vi "GenerateLab.vi"(8 "ROI":T1, 9 "Lighting":u16(ring)=5 items=["Incandescent/tungsten", "Old direct sunlight at noon", "Old daylight", "ICC profile PCS", "Mid-morning daylight", "Daylight, sRGB, Adobe-RGB", "North sky daylight", "Equal energy", "Daylight Fluorescent", "Cool fluorescent", "White Fluorescent", "Warm White Fluorescent", "Daylight Fluorescent", "Lite White Fluorescent", "Daylight fluorescent, D65 simulator", "Sylvania F40, D50 simulator", "Cool White Fluorescent", "Ultralume 50, Philips TL85", "Ultralume 40, Philips TL84", "Ultralume 30, Philips TL83"], 11 "image data":T2) -> (1 "Dimensions":string, 3 "Plots":T3)   [LabVIEW 2020]
uses:
  <vilib>/picture/picture.llb/imagedata.ctl
panel:
  out "b":dbl[](graph)
  out "a":dbl[](graph)
  out "L":dbl[](graph)
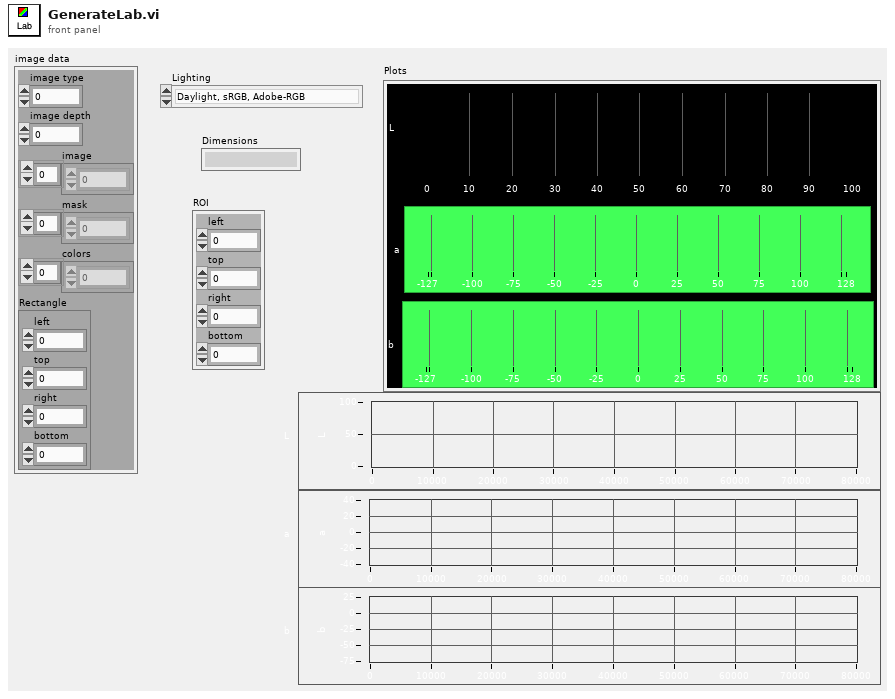
[diagram p1: front panel]
types:
  T1 = cluster{"left":i32, "top":i32, "right":i32, "bottom":i32}
  T2 = typedef "imagedata.ctl" = cluster{"image type":i32, "image depth":i32, "image":u8[], "mask":u8[], "colors":u32[], "Rectangle":cluster{"left":i16, "top":i16, "right":i16, "bottom":i16}}
  T3 = cluster{"L":dbl[], "a":cluster{i32, i32, dbl[]}, "b":cluster{i32, i32, dbl[]}}
  T4 = cluster{dbl[], cluster{i32, i32, dbl[]}, cluster{i32, i32, dbl[]}}
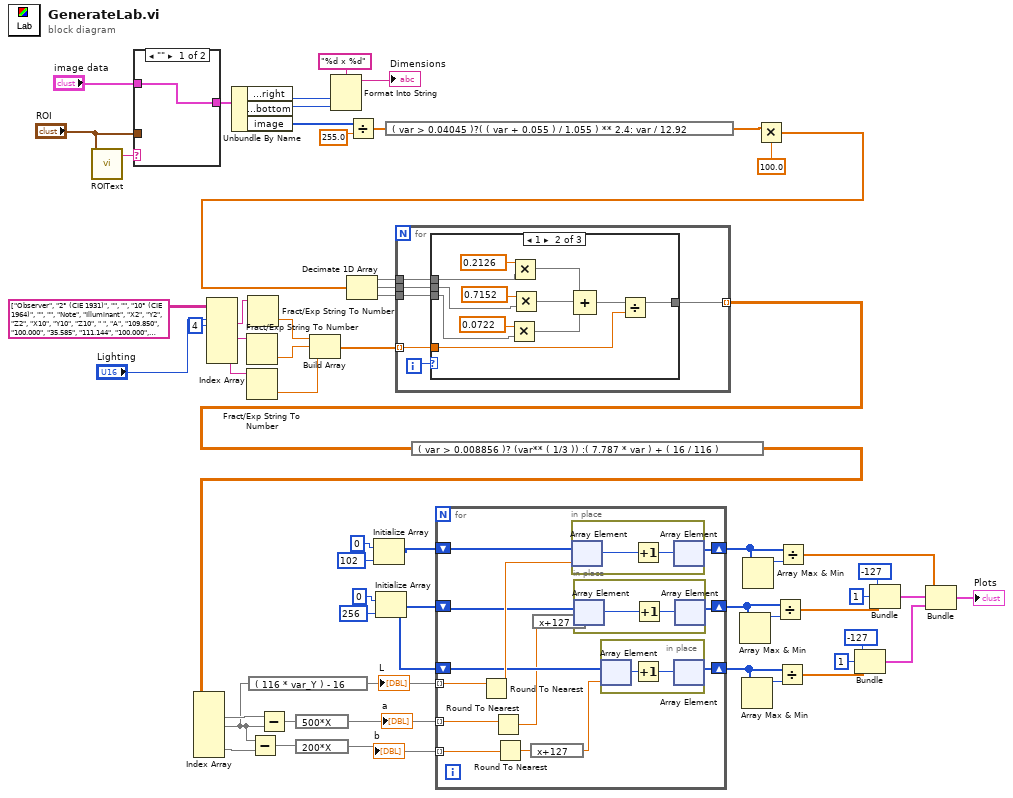
[diagram p0: block diagram]
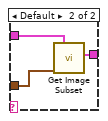
[diagram p2: hidden frame]
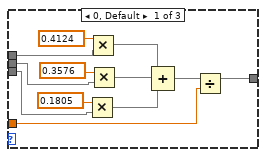
[diagram p3: hidden frame]
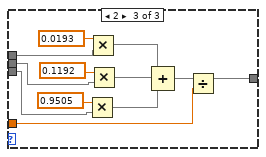
[diagram p4: hidden frame]
diagram:
  n1 = call "ROIText.vi"("ROI"="ROI") -> ("r"=w1:string)  [unwired: 7 in, 3 out]
  n2 = case shown="\"\"" w1 {
    tunnel: "image data" -> [w60 w63]
    tunnel: [w60 w62] -> w3
    tunnel: "ROI" -> [_ w61]
    frame "" {
    }
    frame Default {
      n3 = call <vilib>:"Get Image Subset.vi"("subset rect"=w61, "image data"=w63) -> ("image subset"=w62:T2)  [unwired: 4 in, 1 out]
    }
  }
  n4 = Index Array(array=string[][] [["Observer", "2° (CIE 1931)", "", "", "10° (CIE 1964)", "", "", "Note"], ["Illuminant", "X2", "Y2", "Z2", "X10", "Y10", "Z10", " "], ["A", "109.850", "100.000", "35.585", "111.144", "100.000", "35.200", "Incandescent/tungsten"], ["B", "99.0927", "100.000", "85.313", "99.178;", "100.000", "84.3493", "Old direct sunlight at noon"], ["C", "98.074", "100.000", "118.232", "97.285", "100.000", "116.145", "Old daylight"], ["D50", "96.422", "100.000", "82.521", "96.720", "100.000", "81.427", "ICC profile PCS"], ["D55", "95.682", "100.000", "92.149", "95.799", "100.000", "90.926", "Mid-morning daylight"], ["D65", "95.047", "100.000", "108.883", "94.811", "100.000", "107.304", "Daylight, sRGB, Adobe-RGB"], ["D75", "94.972", "100.000", "122.638", "94.416", "100.000", "120.641", "North sky daylight"], ["E", "100.000", "100.000", "100.000", "100.000", "100.000", "100.000", "Equal energy"], ["F1", "92.834", "100.000", "103.665", "94.791", "100.000", "103.191", "Daylight Fluorescent"], ["F2", "99.187", "100.000", "67.395", "103.280", "100.000", "69.026", "Cool fluorescent"], ["F3", "103.754", "100.000", "49.861", "108.968", "100.000", "51.965", "White Fluorescent"], ["F4", "109.147", "100.000", "38.813", "114.961", "100.000", "40.963", "Warm White Fluorescent"], ["F5", "90.872", "100.000", "98.723", "93.369", "100.000", "98.636", "Daylight Fluorescent"], ["F6", "97.309", "100.000", "60.191", "102.148", "100.000", "62.074", "Lite White Fluorescent"], ["F7", "95.044", "100.000", "108.755", "95.792", "100.000", "107.687", "Daylight fluorescent, D65 simulator"], ["F8", "96.413", "100.000", "82.333", "97.115", "100.000", "81.135", "Sylvania F40, D50 simulator"], ["F9", "100.365", "100.000", "67.868", "102.116", "100.000", "67.826", "Cool White Fluorescent"], ["F10", "96.174", "100.000", "81.712", "99.001", "100.000", "83.134", "Ultralume 50, Philips TL85"], ["F11", "100.966", "100.000", "64.370", "103.866", "100.000", "65.627", "Ultralume 40, Philips TL84"], ["F12", "108.046", "100.000", "39.228", "111.428", "100.000", "40.353", "Ultralume 30, Philips TL83"]] ("Table Control"), index (row) #1="Lighting", index (col) #1=4 ("index (col)")) -> (element #1=w16:string, element #2=w15:string, element #3=w14:string)  [unwired: 4 in]
  n5 = Unbundle By Name(w3) -> ("Rectangle.right"=w20:i16, "Rectangle.bottom"=w19:i16, "image"=w41:u8[])
  n6 = Fract/Exp String To Number(string=w15) -> (number=w10:dbl)  [unwired: 3 in, 1 out]
  n7 = Fract/Exp String To Number(string=w14) -> (number=w9:dbl)  [unwired: 3 in, 1 out]
  n8 = Fract/Exp String To Number(string=w16) -> (number=w11:dbl)  [unwired: 3 in, 1 out]
  n9 = Build Array(w11, w10, w9) -> (w8:dbl[])
  n10 = Format Into String(format string="%d x %d", w20, w19) -> (resulting string=→"Dimensions":string)  [unwired: 2 in, 1 out]
  n11 = Divide(x=w41, y=255.0) -> (x/y=w58:dbl[])
  n12 = Initialize Array(u32 0, 102 ("dimension size")) -> (w38:u32[])
  n13 = Initialize Array(u32 0, 256 ("dimension size")) -> (w45:u32[])
  n14 = expression code="( var > 0.04045 )?( ( var + 0.055 ) / 1.055 ) ** 2.4: var / 12.92"(w58) -> (w43:dbl[])
  n15 = Multiply(x=w43, y=100.0) -> (x*y=w42:dbl[])
  n16 = Decimate 1D Array(w42) -> (w57:dbl[], w56:dbl[], w55:dbl[])
  n17 = for {
    tunnel: w57 -> [w68]
    tunnel: w56 -> [w67]
    tunnel: w55 -> [w66]
    tunnel: [w65] -> w54 mode=indexing
    tunnel: w8 -> [w64] mode=indexing
    i -> [w69]
    n18 = case shown="1" w69 {
      tunnel: w68 -> [w80 w92 w104]
      tunnel: w67 -> [w79 w91 w103]
      tunnel: w66 -> [w78 w90 w102]
      tunnel: [w71 w83 w95] -> w65
      tunnel: w64 -> [w70 w82 w94]
      frame 0, Default {
        n19 = Multiply(x=0.1805, y=w78) -> (x*y=w73:dbl[])
        n20 = Multiply(x=0.4124, y=w80) -> (x*y=w74:dbl[])
        n21 = Multiply(x=0.3576, y=w79) -> (x*y=w75:dbl[])
        n22 = Compound Arithmetic op=ADD(w74, w75, w73) -> (w72:dbl[])
        n23 = Divide(x=w72, y=w70) -> (x/y=w71:dbl[])
      }
      frame 1 {
        n24 = Multiply(x=0.0722, y=w90) -> (x*y=w85:dbl[])
        n25 = Multiply(x=0.2126, y=w92) -> (x*y=w86:dbl[])
        n26 = Multiply(x=0.7152, y=w91) -> (x*y=w87:dbl[])
        n27 = Compound Arithmetic op=ADD(w86, w87, w85) -> (w84:dbl[])
        n28 = Divide(x=w84, y=w82) -> (x/y=w83:dbl[])
      }
      frame 2 {
        n29 = Multiply(x=0.9505, y=w102) -> (x*y=w97:dbl[])
        n30 = Multiply(x=0.0193, y=w104) -> (x*y=w98:dbl[])
        n31 = Multiply(x=0.1192, y=w103) -> (x*y=w99:dbl[])
        n32 = Compound Arithmetic op=ADD(w98, w99, w97) -> (w96:dbl[])
        n33 = Divide(x=w96, y=w94) -> (x/y=w95:dbl[])
      }
    }
  }
  n34 = expression code="( var > 0.008856 )? (var** ( 1/3 )) :( 7.787 * var ) + ( 16 / 116 )"(w54) -> (w53:dbl[][])
  n35 = Index Array(array=w53) -> (element #1=w52:dbl[], element #2=w50:dbl[], element #3=w51:dbl[])  [unwired: 6 in]
  n36 = expression code="( 116 * var_Y ) - 16"(w50) -> (w7:dbl[])
  "L" <- w7
  n37 = Subtract(x=w50, y=w51) -> (x-y=w48:dbl[])
  n38 = Subtract(x=w52, y=w50) -> (x-y=w49:dbl[])
  n39 = expression code="500*X"(w49) -> (w5:dbl[])
  "a" <- w5
  n40 = expression code="200*X"(w48) -> (w6:dbl[])
  "b" <- w6
  n41 = for {
    shift-right: [w117] -> w36
    shift-left: w38 -> [w119]
    shift-right: [w114] -> w34
    shift-left: w45 -> [w115]
    shift-right: [w113] -> w32
    shift-left: w45 -> [w116]
    tunnel: w7 -> [w108] mode=indexing
    tunnel: w5 -> [w107] mode=indexing
    tunnel: w6 -> [w106] mode=indexing
    n42 = Round To Nearest(number=w108) -> (nearest integer value=w118:dbl)
    n43 = Round To Nearest(number=w107) -> (nearest integer value=w111:dbl)
    n44 = Round To Nearest(number=w106) -> (nearest integer value=w112:dbl)
    n45 = expression code="x+127"(w112) -> (w109:dbl)
    n46 = expression code="x+127"(w111) -> (w110:dbl)
    n47 = in-place {
      n48 = in-place-array #1(w119, w118) -> (w125:u32)
      n49 = Increment(x=w125) -> (x+1=w124:u32)
      n50 = in-place-array #1(w124) -> (w117:u32[])  [unwired: 1 out]
    }
    n51 = in-place {
      n52 = in-place-array #2(w115, w110) -> (w123:u32)
      n53 = Increment(x=w123) -> (x+1=w122:u32)
      n54 = in-place-array #2(w122) -> (w114:u32[])  [unwired: 1 out]
    }
    n55 = in-place {
      n56 = in-place-array #3(w116, w109) -> (w121:u32)
      n57 = Increment(x=w121) -> (x+1=w120:u32)
      n58 = in-place-array #3(w120) -> (w113:u32[])  [unwired: 1 out]
    }
  }
  n59 = Array Max & Min(array=w34) -> (max value=w35:u32)  [unwired: 3 out]
  n60 = Array Max & Min(array=w32) -> (max value=w33:u32)  [unwired: 3 out]
  n61 = Array Max & Min(array=w36) -> (max value=w37:u32)  [unwired: 3 out]
  n62 = Divide(x=w34, y=w35) -> (x/y=w31:dbl[])
  n63 = Divide(x=w32, y=w33) -> (x/y=w26:dbl[])
  n64 = Divide(x=w36, y=w37) -> (x/y=w25:dbl[])
  n65 = Bundle(-127, 1, w26) -> (w23:cluster{i32, i32, dbl[]})  [unwired: 1 in]
  n66 = Bundle(-127, 1, w31) -> (w24:cluster{i32, i32, dbl[]})  [unwired: 1 in]
  n67 = Bundle(w25, w24, w23) -> (→"Plots":T4)  [unwired: 1 in]
